vi "Pre Launch Init.vi"(11 "Signal Acquisition in":refnum<class "Signal Acquisition.lvclass">) -> (0 "error out":errorcluster, 3 "Signal Acquisition out":refnum<class "Signal Acquisition.lvclass">)   [LabVIEW 2022 SP3, in "Signal Acquisition.lvlib" / "Signal Acquisition.lvclass"]
doc: "(<B>Filename</B>: Actor Framework.lvlib:Actor.lvclass:Pre Launch Init.vi)\n\nDefines behavior that occurs after the Launch Actor method is invoked but before the actor's Actor Core method begins running.\n\nThe Pre Launch Init method is guaranteed to finish before the Launch Actor method returns to its caller and before the actor itself receives any messages. Any references that the Pre Launch Init method obtains are guaranteed to have the same lifetime as the actor itself. Any errors that the Pre Launch Init method returns will abort the launch.\n\nBy default, this method does nothing. A descendant class may override it to define behavior."
uses:
  Signal Acquisition.lvclass
  Signal Acquisition.lvclass/Signal Acquisition.ctl
  <vilib>/ActorFramework/Actor/Actor.lvclass
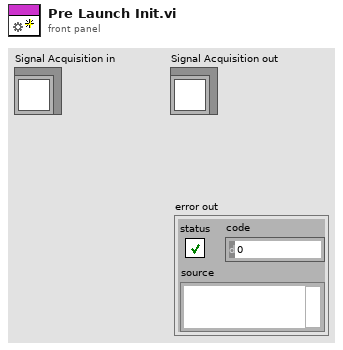
[diagram p1: front panel]
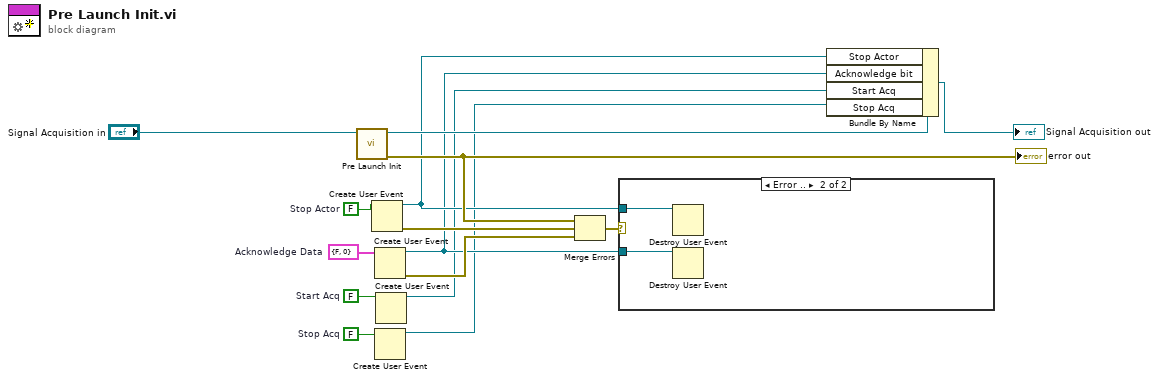
[diagram p0: block diagram]
diagram:
  w1 = FALSE  # Stop Acq
  w4 = FALSE  # Start Acq
  w6 = cluster{"Acknowledge":bool, "Address":u16} {"Acknowledge"=FALSE, "Address"=0}  # Acknowledge Data
  w14 = FALSE  # Stop Actor
  n1 = call-parent "Pre Launch Init.vi"("Actor in"="Signal Acquisition in") -> ("error out"=w10:errorcluster, "Actor out"=w15:refnum<class "Signal Acquisition.lvclass">)  [unwired: 9 in]
  "error out" <- w10
  n2 = Create User Event(user event datatype=w14) -> (user event=w8:refnum<user-event>, error out=w12:errorcluster)  [unwired: 1 in]
  n3 = Create User Event(user event datatype=w6) -> (user event=w5:refnum<user-event>, error out=w7:errorcluster)  [unwired: 1 in]
  n4 = Create User Event(user event datatype=w1) -> (user event=w2:refnum<user-event>)  [unwired: 1 in, 1 out]
  n5 = Create User Event(user event datatype=w4) -> (user event=w3:refnum<user-event>)  [unwired: 1 in, 1 out]
  n6 = Merge Errors(w10, w12, w7) -> (w11:errorcluster)
  n7 = case shown="Error .." w11 {
    tunnel: w8 -> [_ w17]
    tunnel: w5 -> [_ w16]
    frame No Error {
    }
    frame Error {
      n8 = Destroy User Event(user event=w17) -> ()  [unwired: 1 in, 1 out]
      n9 = Destroy User Event(user event=w16) -> ()  [unwired: 1 in, 1 out]
    }
  }
  n10 = Bundle By Name(cluster=w15, "Stop Actor"=w8, "Acknowledge bit"=w5, "Start Acq"=w3, "Stop Acq"=w2) -> (→"Signal Acquisition out":refnum<class "Signal Acquisition.lvclass">)
